vi "1B_AnalyzeAmplitudeRamp.vi"(0 "Trim top":bool, 1 "Ramp Duration ( sec )":dbl=10.0, 3 "DAQ":waveform(dbl)[](array[waveform]), 4 "Input \nWaveform \nRepetitions":i32=4, 5 "Ramp End Pulse Characteristics":T2={"Pulses per Cycle"=4, "Load Resistance (Ohms)"=750.0, "Krec Value"=2, "Recovery Mode (T=Active)"=TRUE, "Amps"=[0.01, 0.008, 0.005, 0.002]} {"Amps" format="%#_6p"}, 6 "Offset Calculation Method":T3=enum."Precise", 7 "Measurement Time Offset ( sec )":dbl=1.2 format="%#.3p", 8 "top trim sec":dbl=1.0, 9 "Tolerance [ A ]":dbl=0.0009 format="%#.3p", 10 "Resampling \nStrength":T4=enum."4", 12 "Smoothing Strength":T5=enum."50") -> (11 "size(s)":i32, 13 "P1 mean error [ A ]":dbl format="%#.0p", 14 "Trimmed Elapsed time from Active Stim ( sec )":dbl[](array[numeric])=[1.8767312026320724, 2.978631206395221, 4.068465751042822, 5.166899951203959, 6.281533743458567, 7.396964385960018, 8.492272259914898, 9.593095214062487, 10.689171075006016] format="%#.1g", 15 "P1":cluster{"Target":dbl[], "Measured":dbl[]} {"Measured" format="%#.1p"; "Target" format="%#.1p"}, 17 "P2":cluster{"Target":dbl[], "Measured":dbl[]} {"Measured" format="%#.1p"; "Target" format="%#.1p"}, 18 "P3":cluster{"Target":dbl[], "Measured":dbl[]} {"Measured" format="%#.1p"; "Target" format="%#.1p"}, 19 "P4":cluster{"Target":dbl[], "Measured":dbl[]} {"Measured" format="%#.1p"; "Target" format="%#.1p"})   [LabVIEW 2010]
uses:
  FilterStrength.ctl
  1B_Resample Strength.ctl
  1B_Offset Calculation Method.ctl
panel:
  out "Measured Frequency":dbl[](array[numeric]) format="%#.1p"
  out "Target Stim Currents f (time) [ A ]":dbl[][](array[numeric]) format="%#.1p"
  out "Calculated Waveform Parameters":T1(array[cluster])=[{"Stim Amplitude"=[0.001890808904666845, 0.0015063789218088246, 0.0009380786181013236, 0.00038046379628492905], "Stim Pulse Width"=[0.00049872, 0.0005983200000000001, 0.0006981600000000001, 0.0007968000000000001], "Interphase Delay"=[0.00017448000000000002, 0.00014808000000000003, 0.00014064, 0.00014184], "Recovery PW"=[1.8720000000000004e-05, 2.9760000000000003e-05, 4.08e-05, 0.00012888000000000003], "Recovery Holdoff"=[0.0, 0.0, 0.0, 0.0], "Avg CBC Width"=6.0240000000000006e-05, "Frequency"=65.10552303172982, "Avg. CBC Holdoff"=0.0, "Recovery Amplitude"=[-0.00048744302134257083, -0.0003935399321504205, -0.00027207913147701227, -0.00011775952554436959]}, {"Stim Amplitude"=[0.0030797504682826674, 0.0024596490036145006, 0.001538178203417415, 0.0006198428888048686], "Stim Pulse Width"=[0.00050016, 0.0006000000000000001, 0.0006996000000000001, 0.0007989600000000001], "Interphase Delay"=[0.00019584000000000002, 0.00015216, 0.00014808000000000003, 0.00014448000000000003], "Recovery PW"=[5.640000000000001e-05, 4.1280000000000005e-05, 3.792e-05, 9.192000000000001e-05], "Recovery Holdoff"=[0.0, 0.0, 0.0, 0.0], "Avg CBC Width"=6.168e-05, "Frequency"=65.10552303172982, "Avg. CBC Holdoff"=0.0, "Recovery Amplitude"=[-0.0007718366356821519, -0.0006280510303097946, -0.0003929174147049414, -0.00017931823402160378]}, {"Stim Amplitude"=[0.00425836078038066, 0.0034003104060010875, 0.002128213626924414, 0.0008495657201374633], "Stim Pulse Width"=[0.00050016, 0.0006000000000000001, 0.0006998400000000001, 0.0007984800000000001], "Interphase Delay"=[0.00014808000000000003, 0.00014472, 0.00015456, 0.00014592], "Recovery PW"=[2.6880000000000004e-05, 6.816000000000001e-05, 7.560000000000001e-05, 0.00018216000000000003], "Recovery Holdoff"=[0.0, 0.0, 0.0, 0.0], "Avg CBC Width"=6.336e-05, "Frequency"=65.11501916986163, "Avg. CBC Holdoff"=0.0, "Recovery Amplitude"=[-0.0010502199185027236, -0.0008674001731176454, -0.0005418286534561375, -0.0002442329941597939]}, {"Stim Amplitude"=[0.005437516859384138, 0.004348103594760739, 0.0027220760954958993, 0.001094712379568853], "Stim Pulse Width"=[0.0005008800000000001, 0.0006007200000000001, 0.0007005600000000001, 0.0008006400000000001], "Interphase Delay"=[0.00014664000000000002, 0.00014736000000000003, 0.00014616000000000002, 0.00014208000000000002], "Recovery PW"=[0.00031656, 0.0018816000000000002, 5.208000000000001e-05, 0.00027312], "Recovery Holdoff"=[0.0, 0.0, 0.0, 0.0], "Avg CBC Width"=6.144000000000001e-05, "Frequency"=65.10009791054725, "Avg. CBC Holdoff"=0.0, "Recovery Amplitude"=[-0.0013432467878205132, -0.0010796594394815965, -0.0006767447519008667, -0.00029349318592438106]}, {"Stim Amplitude"=[0.006592546587772567, 0.005269472904232999, 0.003284228362533635, 0.0013074430142210364], "Stim Pulse Width"=[0.0005006400000000001, 0.00060024, 0.0006996000000000001, 0.0008001600000000001], "Interphase Delay"=[0.0001464, 0.0001452, 0.00014568000000000003, 0.00014256000000000002], "Recovery PW"=[0.0017726400000000002, 0.00237072, 0.00048888, 7.200000000000002e-05], "Recovery Holdoff"=[0.0, 0.0, 0.0, 0.0], "Avg CBC Width"=6.240000000000001e-05, "Frequency"=65.11501916986163, "Avg. CBC Holdoff"=0.0, "Recovery Amplitude"=[-0.001635865189213957, -0.0013173178937903045, -0.0008247288460378789, -0.00035244320537638715]}, {"Stim Amplitude"=[0.007901755320384868, 0.006319564654557489, 0.0039462625480513195, 0.0015731927391993445], "Stim Pulse Width"=[0.0005011200000000001, 0.0006004800000000001, 0.0007005600000000001, 0.0008006400000000001], "Interphase Delay"=[0.0001464, 0.00014472, 0.00014592, 0.00014280000000000003], "Recovery PW"=[0.0019701600000000003, 0.0016507200000000003, 0.0007920000000000001, 0.00028536], "Recovery Holdoff"=[0.0, 0.0, 0.0, 0.0], "Avg CBC Width"=4.584000000000001e-05, "Frequency"=64.07364881489379, "Avg. CBC Holdoff"=0.0, "Recovery Amplitude"=[-0.0019506339074219588, -0.0015677202401563042, -0.0009701481712415901, -0.0004006686778165441]}, {"Stim Amplitude"=[0.00949197457994598, 0.007583522191622097, 0.00473511751245542, 0.0018793522570743175], "Stim Pulse Width"=[0.0005023200000000001, 0.00060192, 0.0007017600000000001, 0.0008020800000000002], "Interphase Delay"=[0.00014328000000000002, 0.00014232, 0.00014280000000000003, 0.00014136000000000002], "Recovery PW"=[0.0019752000000000003, 0.00237576, 0.0027734400000000003, 0.00042024000000000006], "Recovery Holdoff"=[0.0, 0.0, 0.0, 0.0], "Avg CBC Width"=6.144000000000001e-05, "Frequency"=65.10552303172982, "Avg. CBC Holdoff"=0.0, "Recovery Amplitude"=[-0.0023391325168469765, -0.0018816292913810685, -0.0011615176849564522, -0.00046337320256020916]}, {"Stim Amplitude"=[0.01005855346256491, 0.008032568068756981, 0.005010389532814817, 0.001985679855604283], "Stim Pulse Width"=[0.0005004, 0.0006004800000000001, 0.0007000800000000001, 0.0007999200000000001], "Interphase Delay"=[0.00014712000000000001, 0.00014616000000000002, 0.00014712000000000001, 0.00014544000000000002], "Recovery PW"=[0.00196896, 0.0023702400000000005, 0.00036672000000000007, 0.00021192000000000002], "Recovery Holdoff"=[0.0, 0.0, 0.0, 0.0], "Avg CBC Width"=6.192e-05, "Frequency"=65.09874177151903, "Avg. CBC Holdoff"=0.0, "Recovery Amplitude"=[-0.002491351211256549, -0.002006642401177291, -0.0012414179547553478, -0.0005219615253170457]}, {"Stim Amplitude"=[0.010071089713755919, 0.010071149998049042, 0.008036154487546165, 0.005016696740922397], "Stim Pulse Width"=[0.0004982400000000001, 0.0005030400000000001, 0.00060672, 0.0007128000000000001], "Interphase Delay"=[0.013344480000000002, 0.00014064, 0.00013296000000000003, 0.00012336], "Recovery PW"=[5.520000000000001e-05, 0.00197904, 0.0023904000000000004, 0.0028008000000000004], "Recovery Holdoff"=[0.0, 0.0, 0.0, 0.0], "Avg CBC Width"=3.0480000000000003e-05, "Frequency"=97.75706197015671, "Avg. CBC Holdoff"=0.0, "Recovery Amplitude"=[-0.004708942602105241, -0.0024890476595770365, -0.0019978481861519263, -0.0012320418296574223]}] {"Frequency" format="%#.3p"; "Avg CBC Width" format="%#_6p"; "Avg. CBC Holdoff" format="%#_6p"; "Stim Pulse Width" format="%#.3p"; "Interphase Delay" format="%#.3p"; "Recovery PW" format="%#_6p"; "Recovery Holdoff" format="%#.3p"; "Stim Amplitude" format="%#.3p"; "Recovery Amplitude" format="%#_6p"}
  # "Open subVI \"1B_AnalyzeAmplitudeRamp_LimitsGraph.vi\" to view results."
  # "e.g. 1.2"
  # "Tip: Select \"Simple\" if \"Precise\" cannot mesure offset"
  # "Tip: Decreasing Repetitions may yield better results"
  # "End -->"
  # "Enter Target Current\nfor each in array below"
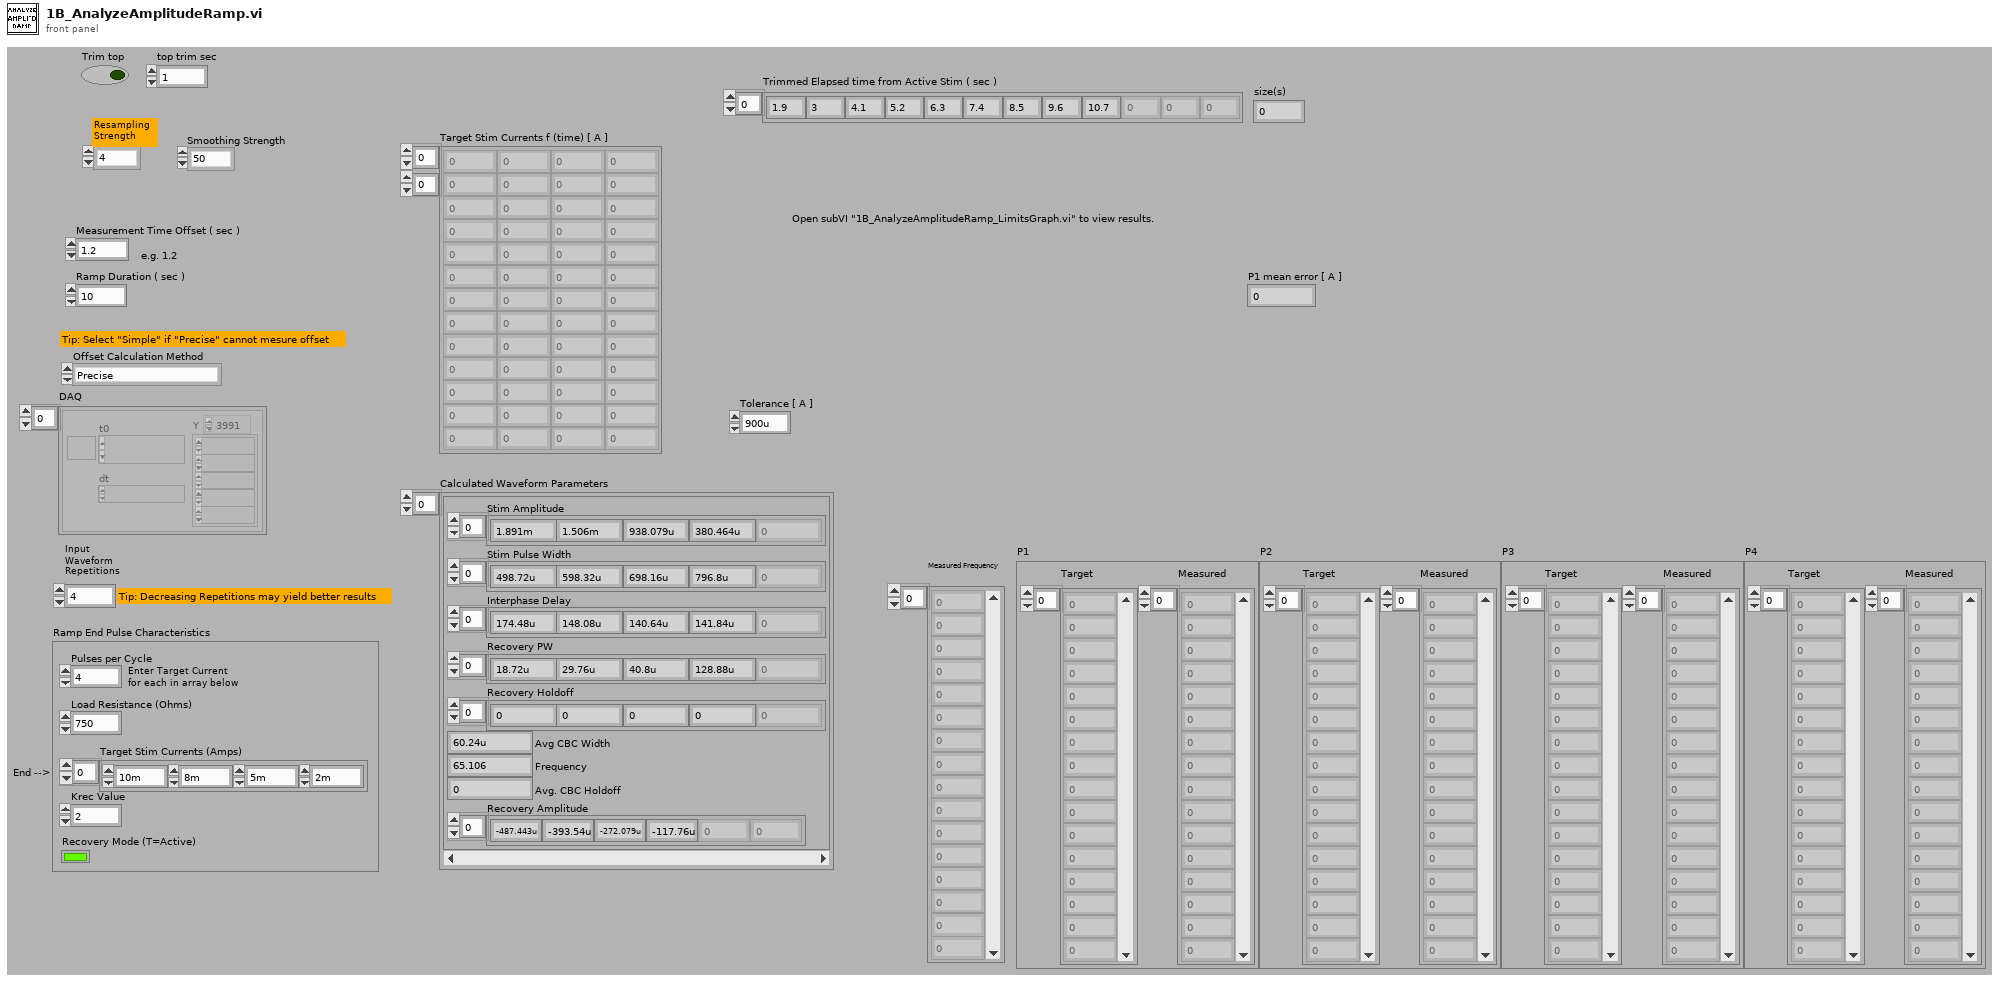
[diagram p1: front panel]
types:
  T1 = cluster{"Stim Amplitude":dbl[], "Stim Pulse Width":dbl[], "Interphase Delay":dbl[], "Recovery PW":dbl[], "Recovery Holdoff":dbl[], "Avg CBC Width":dbl, "Frequency":dbl, "Avg. CBC Holdoff":dbl, "Recovery Amplitude":dbl[]}[]
  T2 = cluster{"Pulses per Cycle":i32, "Load Resistance (Ohms)":dbl, "Krec Value":i32, "Recovery Mode (T=Active)":bool, "Amps":dbl[]}
  T3 = typedef "1B_Offset Calculation Method.ctl" = enum16{"Obsolete", "Precise", "Simple"}
  T4 = typedef "1B_Resample Strength.ctl" = enum16{"Off", "2", "4", "8", "16", "32"}
  T5 = typedef "FilterStrength.ctl" = enum16{"Off", "10", "20", "50", "100", "200", "500", "1000"}
  T6 = cluster{"Stim Amplitude":dbl[], "Stim Pulse Width":dbl[], "Interphase Delay":dbl[], "Recovery PW":dbl[], "Recovery Holdoff":dbl[], "Avg CBC Width":dbl, "Frequency":dbl, "Avg. CBC Holdoff":dbl, "Recovery Amplitude":dbl[]}
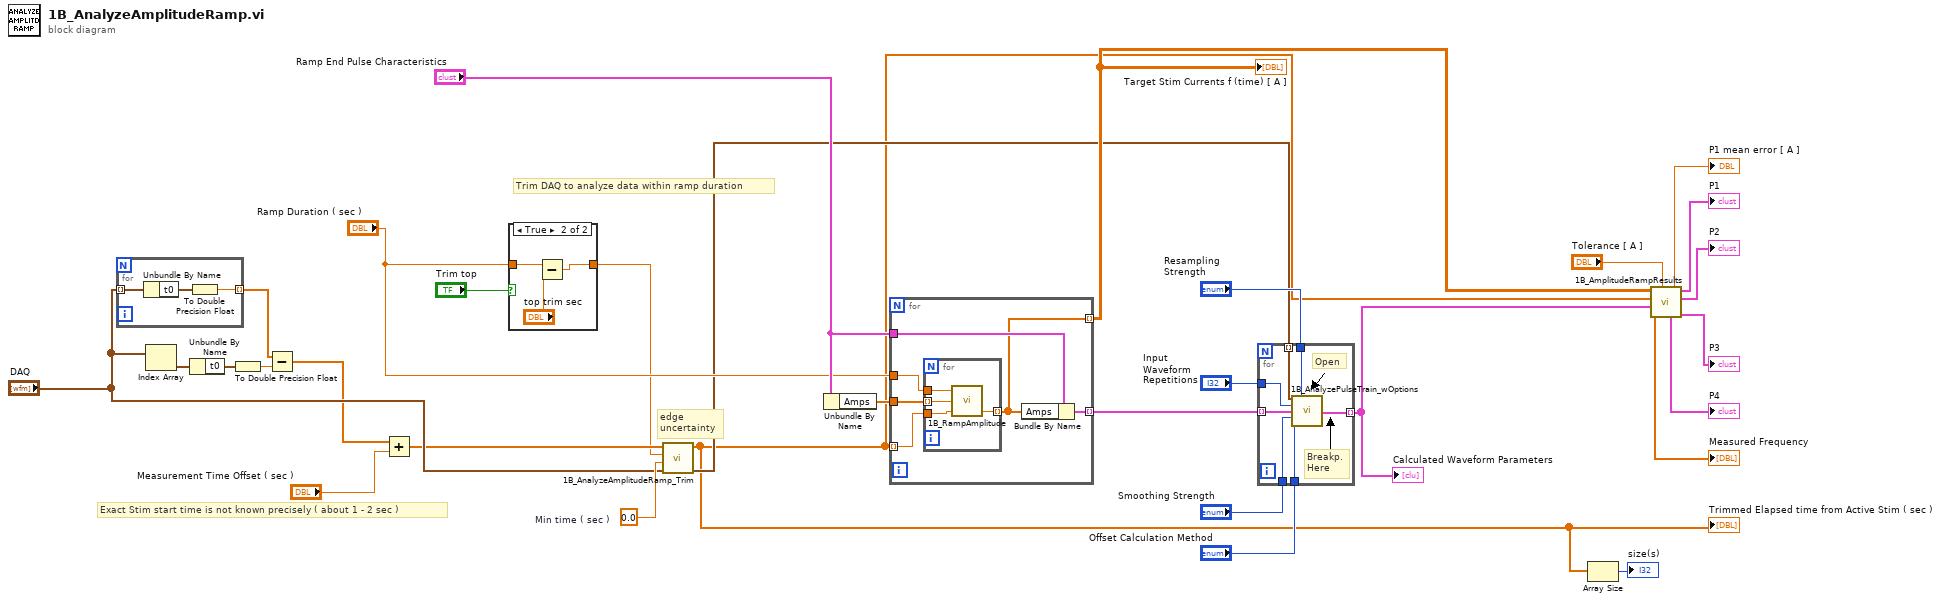
[diagram p0: block diagram]
diagram:
  w21 = 0.0  # Min time ( sec )
  # "edge\nuncertainty"
  # "Exact Stim start time is not known precisely ( about 1 - 2 sec )"
  # "Trim DAQ to analyze data within ramp duration"
  n1 = for {
    tunnel: "DAQ" -> [w34] mode=indexing
    tunnel: [w32] -> w13 mode=indexing
    n2 = Unbundle By Name(w34) -> ("t0"=w33:timestamp)
    n3 = To Double Precision Float(number=w33) -> (double precision float=w32:dbl)
  }
  n4 = Index Array(array="DAQ") -> (element=w12:waveform(dbl))  [unwired: 1 in]
  n5 = Unbundle By Name(w12) -> ("t0"=w11:timestamp)
  n6 = To Double Precision Float(number=w11) -> (double precision float=w14:dbl)
  n7 = Subtract(x=w13, y=w14) -> (x-y=w9:dbl[])
  n8 = Add(x=w9, y="Measurement Time Offset ( sec )") -> (x+y=w8:dbl[])
  n9 = case shown="True" "Trim top" {
    tunnel: "Ramp Duration ( sec )" -> [w35 w38]
    tunnel: [w35 w37] -> w7
    frame False {
    }
    frame True {
      n10 = Subtract(x=w38, y="top trim sec") -> (x-y=w37:dbl)
    }
  }
  n11 = call "1B_AnalyzeAmplitudeRamp_Trim.vi"("Array"="DAQ", "Min time ( sec )"=w21, "Max Time ( sec )"=w7, "Elapsed time from Active Stim ( sec )"=w8) -> ("Array out"=w20:waveform(dbl)[], "Elapsed time from Active Stim ( sec ) out"=w3:dbl[])  [unwired: 6 in]
  "Trimmed Elapsed time from Active Stim ( sec )" <- w3
  n12 = Unbundle By Name("Ramp End Pulse Characteristics") -> ("Amps"=w27:dbl[])
  n13 = for {
    tunnel: w3 -> [w43] mode=indexing
    tunnel: w27 -> [w44]
    tunnel: "Ramp Duration ( sec )" -> [w42]
    tunnel: "Ramp End Pulse Characteristics" -> [w41]
    tunnel: [w40] -> w25 mode=indexing
    tunnel: [w39] -> w24 mode=indexing
    n14 = for {
      tunnel: w44 -> [w48] mode=indexing
      tunnel: w43 -> [w47]
      tunnel: w42 -> [w46]
      tunnel: [w45] -> w39 mode=indexing
      n15 = call "1B_RampAmplitude.vi"("Elapsed time from Active Stim ( sec )"=w47, "End-Ramp Amplitude ( mA )"=w48, "Ramp Duration ( sec )"=w46) -> ("Expected Amplitude at time( mA )"=w45:dbl)  [unwired: 2 in]
    }
    n16 = Bundle By Name(cluster=w41, "Amps"=w39) -> (w40:T2)
  }
  "Target Stim Currents f (time) [ A ]" <- w24
  n17 = for {
    tunnel: w20 -> [w55] mode=indexing
    tunnel: "Resampling \nStrength" -> [w54]
    tunnel: "Input \nWaveform \nRepetitions" -> [w53]
    tunnel: "Smoothing Strength" -> [w52]
    tunnel: "Offset Calculation Method" -> [w51]
    tunnel: w25 -> [w50] mode=indexing
    tunnel: [w49] -> w23 mode=indexing
    # "Open"
    # "Breakp.\nHere"
    n18 = call "1B_AnalyzePulseTrain_wOptions.vi"("Waveform In"=w55, "Resampling Strength"=w54, "Repetitions in the Input Waveform"=w53, "Pulse Characteristics"=w50, "Smoothing Strength"=w52, "Offset Calculation Method"=w51) -> ("Waveform Parameters"=w49:T6)  [unwired: 9 out]
  }
  "Calculated Waveform Parameters" <- w23
  n19 = Array Size(array=w3) -> (size(s)=→"size(s)":i32)
  n20 = call "1B_AmplitudeRampResults.vi"("Tolerance [ A ]"="Tolerance [ A ]", "Array 2"=w23, "Time"=w3, "Array 3"=w24) -> ("Cluster 2"=→"P3":cluster{dbl[], dbl[]}, "Cluster 3"=→"P2":cluster{dbl[], dbl[]}, "Cluster 4"=→"P1":cluster{dbl[], dbl[]}, "Cluster"=→"P4":cluster{dbl[], dbl[]}, "P1 mean error [ A ]"=→"P1 mean error [ A ]":dbl, "Measured Frequency"=→"Measured Frequency":dbl[])  [unwired: 1 in, 1 out]
